vi "DDFL_Controller.vi"(0 "K":dbl[](array[numeric]), 1 "q_ref":dbl[](array[numeric]), 2 "q1":dbl, 3 "q2":dbl, 4 "q3":dbl, 5 "q4":dbl, 6 "v_external":dbl, 7 "K1":dbl, 8 "Collect data ?":bool, 9 "K2":dbl, 10 "Robust Control ?":bool, 11 "K3":dbl, 13 "K4":dbl) -> (16 "u_out":dbl, 17 "v(q)":dbl(graph))   [LabVIEW 2021]
uses:
  <vilib>/Simulation/Shared/_Datatypes/SIM SISO Transfer Function.ctl
  <vilib>/Analysis/baseanly.llb/Real A x B.vi
  <vilib>/Simulation/DiscreteLinear/Implementation/NILVSim Discrete Transfer Function Direct.llb/SIM Discrete Transfer Function Diagram (SISO).vi
  <vilib>/Simulation/ContinuousLinear/Implementation/Shared/SIM Transfer Function Support.llb/SIM TransferFunction Normalize to Buffer.vi
  <vilib>/Simulation/DiscreteLinear/Implementation/Shared/SIM Init Discrete States.vi
  <vilib>/Simulation/DiscreteLinear/Implementation/NILVSim Discrete Transfer Function Direct.llb/SIM Transfer Function Direct core (SISO).vi
  <vilib>/Simulation/ContinuousLinear/Implementation/Shared/SIM Transfer Function Support.llb/SIM TransferFunction Normalize.vi
  <vilib>/Simulation/Implementation/Shared/SIM Polynomials.llb/SIM Remove Zero Coefficients (DBL).vi
  <vilib>/Analysis/Matrix/Numeric/Conversions/Matrix To Array - RM.vi
  <vilib>/Analysis/Matrix/Numeric/Conversions/Array To Matrix - RA2.vi
  <vilib>/Analysis/Matrix/Numeric/Multiply/Multiply - RM,R.vi
  <vilib>/Simulation/Implementation/Shared/SIM Polynomials.llb/SIM Divide Polynomials (DBL).vi
  <vilib>/Simulation/Implementation/Shared/SIM BuildSimErr.vi
  <vilib>/Simulation/Implementation/XNodeFramework/SimXNode/SimX.xnode
  <vilib>/Analysis/Matrix/NI_Matrix.lvlib
  <vilib>/Analysis/NI_AALBase.lvlib
panel:
  out "Etta(q)":dbl(graph)
  out "q1":dbl(graph)
  out "Control input u":dbl(graph)
  out "Gamma(q)":dbl(graph)
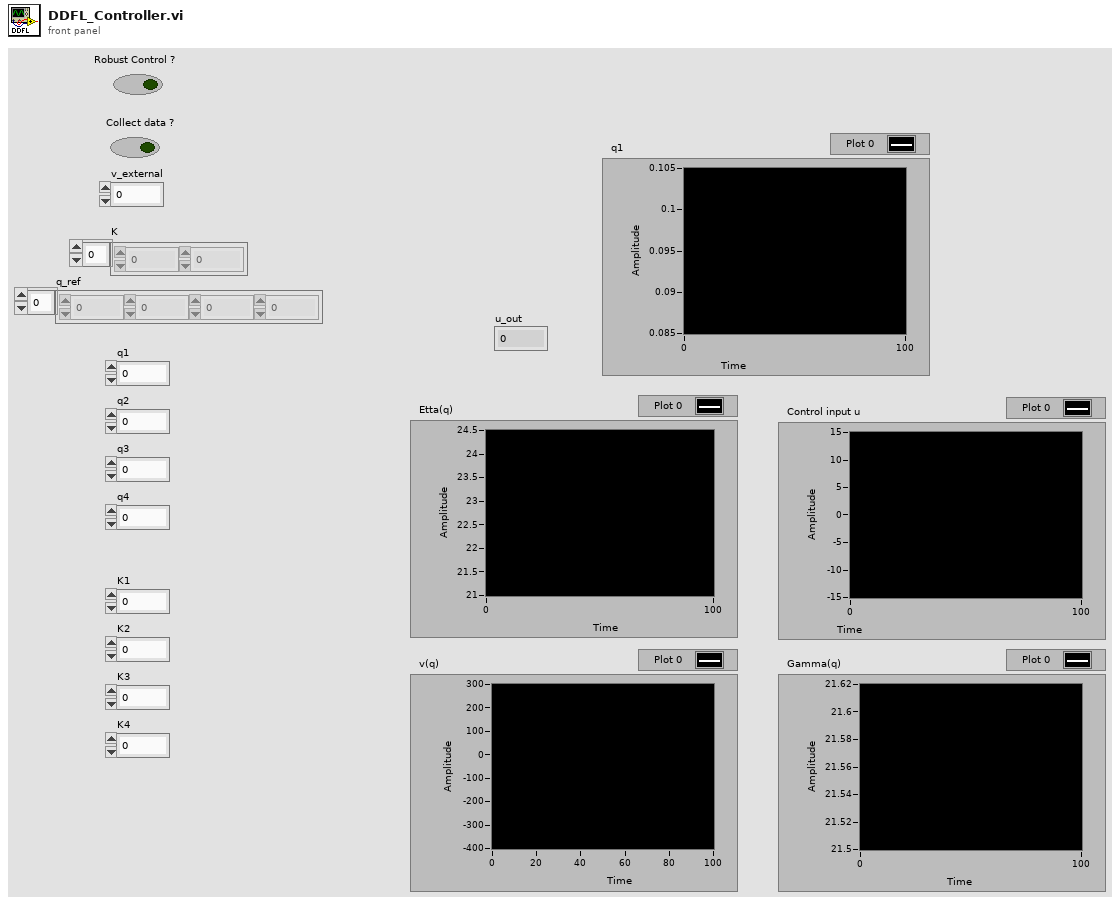
[diagram p1: front panel]
types:
  T1 = typedef "NI_Matrix.lvlib/RealMatrix.ctl" = dbl[][]
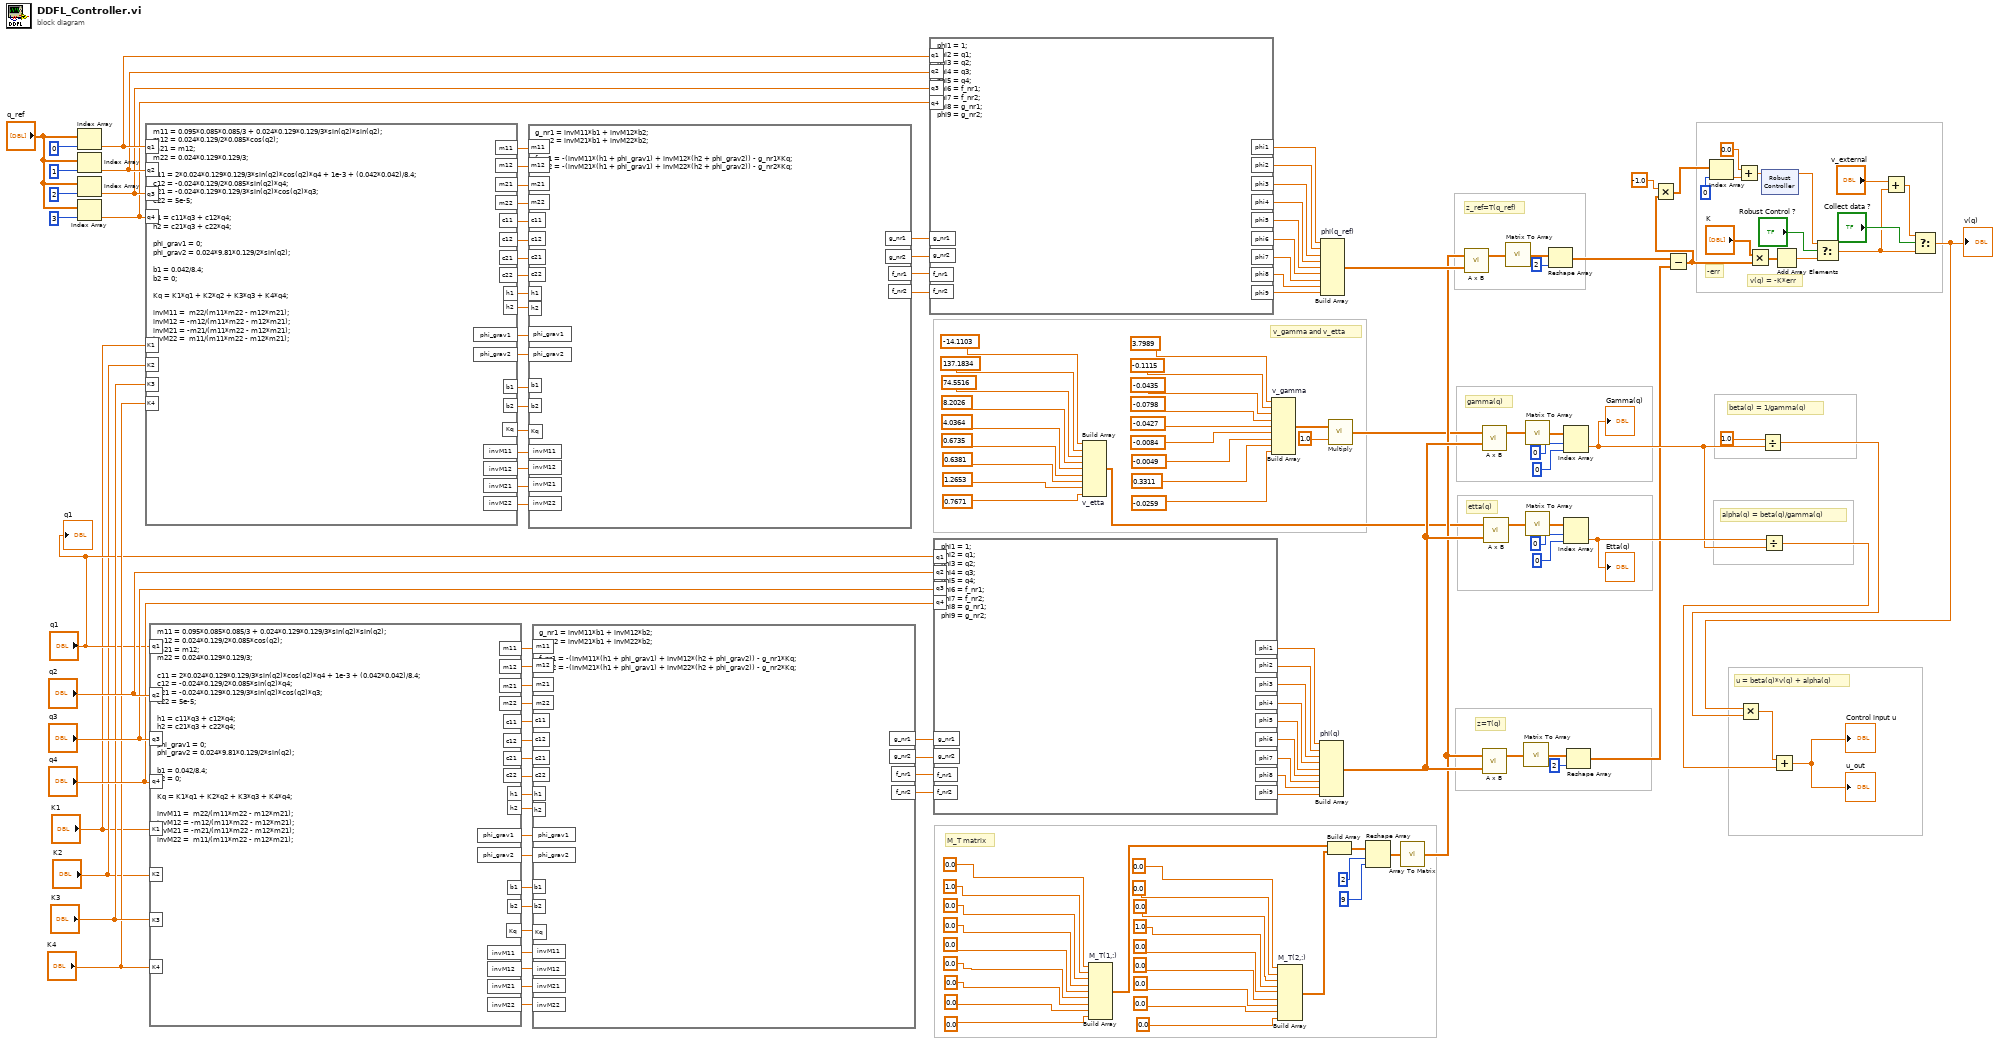
[diagram p0: block diagram]
diagram:
  # "u = beta(q)*v(q) + alpha(q)"
  # "M_T matrix"
  # "v_gamma and v_etta"
  # "alpha(q) = beta(q)/gamma(q)"
  # "beta(q) = 1/gamma(q)"
  # "z_ref=T(q_ref)"
  # "v(q) = -K*err"
  # "-err"
  # "z=T(q)"
  # "etta(q)"
  # "gamma(q)"
  n1 = Index Array(array="q_ref", index=0 ("index 3")) -> (element=w45:dbl)
  n2 = Index Array(array="q_ref", index=1 ("index 4")) -> (element=w43:dbl)
  n3 = Index Array(array="q_ref", index=2 ("index 3")) -> (element=w42:dbl)
  n4 = Index Array(array="q_ref", index=3 ("index 4")) -> (element=w41:dbl)
  n5 = formula code="m11 = 0.095*0.085*0.085/3 + 0.024*0.129*0.129/3*sin(q2)*sin(q2);\nm12 = 0.024*0.129/2*0.085*cos(q2);\nm21 = m12;\nm22 = 0.024*0.129*0.129/3;\n\nc11 = 2*0.024*0.129*0.129/3*sin(q2)*cos(q2)*q4 + 1e-3 + (0.042*0.042)/8.4;\nc12 = -0.024*0.129/2*0.085*sin(q2)*q4;\nc21 = -0.024*0.129*0.129/3*sin(q2)*cos(q2)*q3;\nc22 = 5e-5;\n\nh1 = c11*q3 + c12*q4;\nh2 = c21*q3 + c22*q4;\n\nphi_grav1 = 0;\nphi_grav2 = 0.024*9.81*0.129/2*sin(q2);\n\nb1 = 0.042/8.4;\nb2 = 0;\n\nKq = K1*q1 + K2*q2 + K3*q3 + K4*q4;\n\ninvM11 =  m22/(m11*m22 - m12*m21);\ninvM12 = -m12/(m11*m22 - m12*m21);\ninvM21 = -m21/(m11*m22 - m12*m21);\ninvM22 =  m11/(m11*m22 - m12*m21);"("q1"=w45, "q2"=w43, "q3"=w42, "q4"=w41, "K1"="K1", "K2"="K2", "K3"="K3", "K4"="K4") -> ("m11"=w84:dbl, "m12"=w83:dbl, "m21"=w82:dbl, "m22"=w81:dbl, "c11"=w80:dbl, "c12"=w79:dbl, "c21"=w78:dbl, "c22"=w77:dbl, "h1"=w76:dbl, "h2"=w75:dbl, "phi_grav1"=w74:dbl, "phi_grav2"=w73:dbl, "b1"=w72:dbl, "b2"=w71:dbl, "Kq"=w70:dbl, "invM11"=w69:dbl, "invM12"=w68:dbl, "invM21"=w67:dbl, "invM22"=w66:dbl)
  n6 = formula code="m11 = 0.095*0.085*0.085/3 + 0.024*0.129*0.129/3*sin(q2)*sin(q2);\nm12 = 0.024*0.129/2*0.085*cos(q2);\nm21 = m12;\nm22 = 0.024*0.129*0.129/3;\n\nc11 = 2*0.024*0.129*0.129/3*sin(q2)*cos(q2)*q4 + 1e-3 + (0.042*0.042)/8.4;\nc12 = -0.024*0.129/2*0.085*sin(q2)*q4;\nc21 = -0.024*0.129*0.129/3*sin(q2)*cos(q2)*q3;\nc22 = 5e-5;\n\nh1 = c11*q3 + c12*q4;\nh2 = c21*q3 + c22*q4;\n\nphi_grav1 = 0;\nphi_grav2 = 0.024*9.81*0.129/2*sin(q2);\n\nb1 = 0.042/8.4;\nb2 = 0;\n\nKq = K1*q1 + K2*q2 + K3*q3 + K4*q4;\n\ninvM11 =  m22/(m11*m22 - m12*m21);\ninvM12 = -m12/(m11*m22 - m12*m21);\ninvM21 = -m21/(m11*m22 - m12*m21);\ninvM22 =  m11/(m11*m22 - m12*m21);"("q1"="q1", "q2"="q2", "q3"="q3", "q4"="q4", "K1"="K1", "K2"="K2", "K3"="K3", "K4"="K4") -> ("m11"=w110:dbl, "m12"=w109:dbl, "m21"=w108:dbl, "m22"=w107:dbl, "c11"=w106:dbl, "c12"=w105:dbl, "c21"=w104:dbl, "c22"=w103:dbl, "h1"=w102:dbl, "h2"=w101:dbl, "phi_grav1"=w100:dbl, "phi_grav2"=w99:dbl, "b1"=w98:dbl, "b2"=w97:dbl, "Kq"=w96:dbl, "invM11"=w95:dbl, "invM12"=w94:dbl, "invM21"=w93:dbl, "invM22"=w92:dbl)
  n7 = formula code="g_nr1 = invM11*b1 + invM12*b2;\ng_nr2 = invM21*b1 + invM22*b2;\n\nf_nr1 = -(invM11*(h1 + phi_grav1) + invM12*(h2 + phi_grav2)) - g_nr1*Kq;\nf_nr2 = -(invM21*(h1 + phi_grav1) + invM22*(h2 + phi_grav2)) - g_nr2*Kq;"("m11"=w84, "m12"=w83, "m21"=w82, "m22"=w81, "invM11"=w69, "invM12"=w68, "invM21"=w67, "invM22"=w66, "c11"=w80, "c12"=w79, "c21"=w78, "c22"=w77, "h1"=w76, "h2"=w75, "phi_grav1"=w74, "phi_grav2"=w73, "b1"=w72, "b2"=w71, "Kq"=w70) -> ("g_nr1"=w65:dbl, "g_nr2"=w64:dbl, "f_nr1"=w63:dbl, "f_nr2"=w62:dbl)
  n8 = formula code="g_nr1 = invM11*b1 + invM12*b2;\ng_nr2 = invM21*b1 + invM22*b2;\n\nf_nr1 = -(invM11*(h1 + phi_grav1) + invM12*(h2 + phi_grav2)) - g_nr1*Kq;\nf_nr2 = -(invM21*(h1 + phi_grav1) + invM22*(h2 + phi_grav2)) - g_nr2*Kq;"("m11"=w110, "m12"=w109, "m21"=w108, "m22"=w107, "invM11"=w95, "invM12"=w94, "invM21"=w93, "invM22"=w92, "c11"=w106, "c12"=w105, "c21"=w104, "c22"=w103, "h1"=w102, "h2"=w101, "phi_grav1"=w100, "phi_grav2"=w99, "b1"=w98, "b2"=w97, "Kq"=w96) -> ("g_nr1"=w91:dbl, "g_nr2"=w90:dbl, "f_nr1"=w89:dbl, "f_nr2"=w88:dbl)
  n9 = formula code="phi1 = 1;\nphi2 = q1;\nphi3 = q2;\nphi4 = q3;\nphi5 = q4;\nphi6 = f_nr1;\nphi7 = f_nr2;\nphi8 = g_nr1;\nphi9 = g_nr2;"("q1"=w45, "q2"=w43, "q3"=w42, "q4"=w41, "g_nr1"=w65, "g_nr2"=w64, "f_nr1"=w63, "f_nr2"=w62) -> ("phi1"=w61:dbl, "phi2"=w60:dbl, "phi3"=w59:dbl, "phi4"=w58:dbl, "phi5"=w57:dbl, "phi6"=w56:dbl, "phi7"=w55:dbl, "phi8"=w54:dbl, "phi9"=w53:dbl)
  n10 = formula code="phi1 = 1;\nphi2 = q1;\nphi3 = q2;\nphi4 = q3;\nphi5 = q4;\nphi6 = f_nr1;\nphi7 = f_nr2;\nphi8 = g_nr1;\nphi9 = g_nr2;"("q1"="q1", "q2"="q2", "q3"="q3", "q4"="q4", "g_nr1"=w91, "g_nr2"=w90, "f_nr1"=w89, "f_nr2"=w88) -> ("phi1"=w118:dbl, "phi2"=w117:dbl, "phi3"=w116:dbl, "phi4"=w115:dbl, "phi5"=w114:dbl, "phi6"=w113:dbl, "phi7"=w112:dbl, "phi8"=w20:dbl, "phi9"=w111:dbl)
  n11 = Build Array "v_etta"(-14.1103, 137.1834, 74.5516, 8.2026, 4.0364, 0.6735, 0.6381, 1.2653, 0.7671) -> (w21:T1)
  n12 = Build Array "M_T(1,:)"(0.0, 1.0, 0.0, 0.0, 0.0, 0.0, 0.0, 0.0, 0.0) -> (w124:T1)
  n13 = Build Array "v_gamma"(3.7989, -0.1115, -0.0435, -0.0798, -0.0427, -0.0084, -0.0049, 0.3311, -0.0259) -> (w31:T1)
  n14 = Build Array "M_T(2,:)"(0.0, 0.0, 0.0, 1.0, 0.0, 0.0, 0.0, 0.0, 0.0) -> (w123:T1)
  n15 = Build Array "phi(q)"(w118, w117, w116, w115, w114, w113, w112, w20, w111) -> (w162:T1)
  n16 = Build Array "phi(q_ref)"(w61, w60, w59, w58, w57, w56, w55, w54, w53) -> (w49:T1)
  n17 = Build Array(w124, w123) -> (w122:dbl[][][])
  n18 = call-poly <vilib>:"Multiply.vi"("Real Scalar c"=1.0, "Real Matrix A"=w31) -> ("A * c"=w33:T1)
  n19 = Reshape Array(w122, 2, 9) -> (w119:dbl[][])
  n20 = call-poly <vilib>:"Array To Matrix.vi"("Real 2D Array"=w119) -> ("Real Matrix"=w48:T1)
  n21 = call-poly <vilib>:"A x B.vi"("B"=w49, "A"=w48) -> ("A x B"=w52:T1)  [unwired: 1 out]
  n22 = call-poly <vilib>:"A x B.vi"("B"=w162, "A"=w33) -> ("A x B"=w158:T1)  [unwired: 1 out]
  n23 = call-poly <vilib>:"A x B.vi"("B"=w162, "A"=w48) -> ("A x B"=w154:T1)  [unwired: 1 out]
  n24 = call-poly <vilib>:"A x B.vi"("B"=w162, "A"=w21) -> ("A x B"=w153:T1)  [unwired: 1 out]
  n25 = call-poly <vilib>:"Matrix To Array.vi"("Real Matrix"=w52) -> ("Real 2D Array"=w51:dbl[][])
  n26 = call-poly <vilib>:"Matrix To Array.vi"("Real Matrix"=w154) -> ("Real 2D Array"=w152:dbl[][])
  n27 = call-poly <vilib>:"Matrix To Array.vi"("Real Matrix"=w158) -> ("Real 2D Array"=w161:dbl[][])
  n28 = call-poly <vilib>:"Matrix To Array.vi"("Real Matrix"=w153) -> ("Real 2D Array"=w157:dbl[][])
  n29 = Reshape Array(w51, 2 ("dimension size")) -> (w17:dbl[])
  n30 = Index Array ("Index Array 2")(array=w161, index (row)=0 ("index 3"), index (col)=0 ("index 4")) -> (element=w18:dbl)
  "Gamma(q)" <- w18
  n31 = Index Array ("Index Array 2")(array=w157, index (row)=0 ("index 3"), index (col)=0 ("index 4")) -> (element=w19:dbl)
  "Etta(q)" <- w19
  n32 = Reshape Array(w152, 2 ("dimension size")) -> (w16:dbl[])
  n33 = Subtract(x=w17, y=w16) -> (x-y=w3:dbl[])
  n34 = Multiply(x=-1.0 ("index 3"), y=w3) -> (x*y=w2:dbl[])
  n35 = Index Array ("Index Array 2")(array=w2, index=0 ("index 3")) -> (element=w7:dbl)
  n36 = Add(x=0.0 ("index 3"), y=w7) -> (x+y=w8:dbl)
  n37 = Multiply(x="K", y=w3) -> (x*y=w15:dbl[])
  n38 = Divide(x=1.0, y=w18) -> (x/y=w29:dbl)
  n39 = xnode "Robust Controller"("input u(k)"=w8) -> ("output y(k)"=w11:dbl)  [unwired: 2 in, 1 out]
  n40 = Divide(x=w19, y=w18) -> (x/y=w14:dbl)
  n41 = Add Array Elements(numeric array=w15) -> (sum=w13:dbl)
  n42 = Select ("Select 22")(t=w11, s="Robust Control ?", f=w13) -> (s? t:f=w5:dbl)
  n43 = Add(x="v_external", y=w5) -> (x+y=w4:dbl)
  n44 = Select ("Select 22")(t=w4, s="Collect data ?", f=w5) -> (s? t:f=w25:dbl)
  "v(q)" <- w25
  n45 = Multiply(x=w25, y=w29) -> (x*y=w28:dbl)
  n46 = Add(x=w28, y=w14) -> (x+y=→"u_out" →"Control input u":dbl)
  "q1" <- "q1"
